vi "Do Action.vi"(7 "Self Enqueuer":refnum<class "Message Enqueuer.lvclass">, 8 "error in (no error)":errorcluster, 11 "Change Column Header in":refnum<class "Change Column Header.lvclass">) -> (0 "error out":errorcluster)   [LabVIEW 2016, in "Assert API Components.lvlib" / "Assert Display.lvlib" / "Main Display.lvlib" / "Change Column Header.lvclass"]
uses:
  Change Column Header.lvclass
  <vilib>/ActorFramework/Message Enqueuer/Message Enqueuer.lvclass
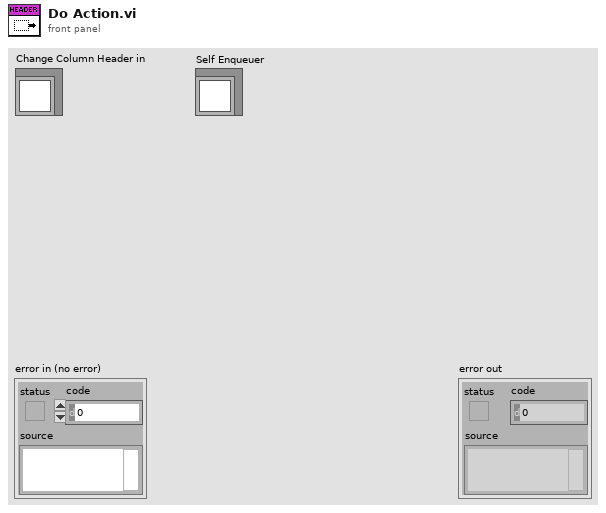
[diagram p1: front panel]
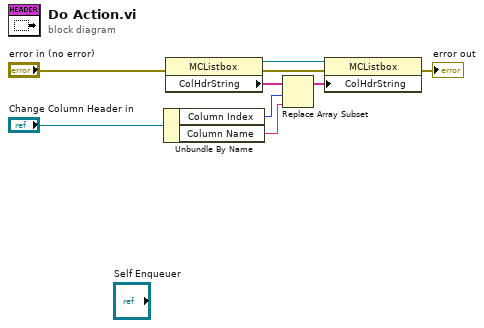
[diagram p0: block diagram]
diagram:
  n1 = Unbundle By Name("Change Column Header in") -> ("Column Index"=w8:i32, "Column Name"=w7:string)
  n2 = property class="MCListbox"(error in="error in (no error)") -> (reference=w1:refnum<vi>, reference out=w6:refnum<vi>, error out=w5:errorcluster, "ColHdrString"=w9:string[])
  n3 = Replace Array Subset(array=w9, new element=w7, index=w8) -> (w4:string[])
  n4 = property class="MCListbox"(reference=w6, error in=w5, "ColHdrString"=w4) -> (error out=→"error out":errorcluster)  [unwired: 1 out]
